vi "JOY_NORM.vi"(9 "Deadband":dbl, 11 "Joy Input":dbl) -> (3 "Joy Output":dbl)   [LabVIEW 2019]
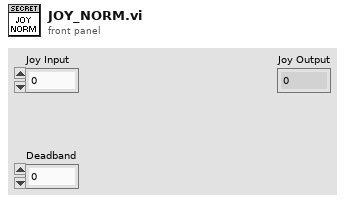
[diagram p1: front panel]
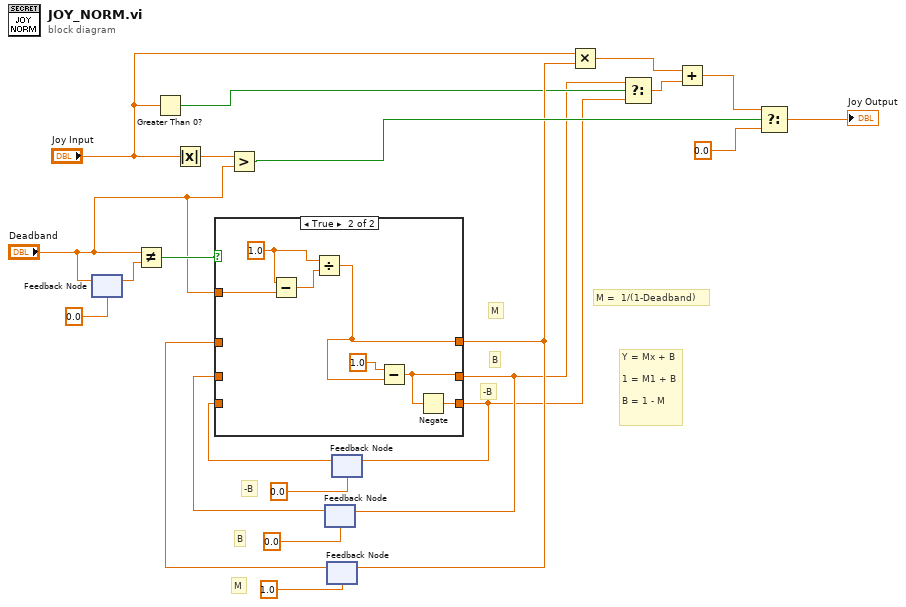
[diagram p0: block diagram]
diagram:
  # "-B"
  # "-B"
  # "M =  1/(1-Deadband)"
  # "Y = Mx + B\n\n1 = M1 + B\n\nB = 1 - M"
  # "M"
  # "B"
  # "B"
  # "M"
  n1 = feedback-in #1("Deadband") -> ()
  n2 = feedback #1(0.0 ("Deadband")) -> (w22:dbl)
  n3 = Not Equal?(x="Deadband", y=w22) -> (x != y?=w20:bool)
  n4 = Greater Than 0?(x="Joy Input") -> (x > 0?=w6:bool)
  n5 = Absolute Value(x="Joy Input") -> (abs(x)=w15:dbl)
  n6 = Greater?(x=w15, y="Deadband") -> (0:w13:bool)
  n7 = feedback #2(0.0 ("Deadband")) -> (w17:dbl)
  n8 = feedback #3(1.0 ("Deadband")) -> (w16:dbl)
  n9 = feedback #4(0.0 ("Deadband")) -> (w2:dbl)
  n10 = case shown="True" w20 {
    tunnel: w17 -> [w24 _]
    tunnel: [w24 w27] -> w5
    tunnel: w16 -> [w25 _]
    tunnel: [w25 w29] -> w11
    tunnel: "Deadband" -> [_ w30]
    tunnel: [w23 w26] -> w1
    tunnel: w2 -> [w23 _]
    frame False {
    }
    frame True {
      w31 = 1.0 ("x")
      n11 = Subtract(x=w31, y=w30) -> (x-y=w32:dbl)
      n12 = Divide(x=w31, y=w32) -> (x/y=w29:dbl)
      n13 = Subtract(x=1.0, y=w29) -> (x-y=w27:dbl)
      n14 = Negate(x=w27) -> (-x=w26:dbl)
    }
  }
  n15 = feedback-in #2(w5) -> ()
  n16 = feedback-in #3(w11) -> ()
  n17 = feedback-in #4(w1) -> ()
  n18 = Multiply(x="Joy Input", y=w11) -> (x*y=w10:dbl)
  n19 = Select(t=w5, s=w6, f=w1) -> (s? t:f=w8:dbl)
  n20 = Add(x=w10, y=w8) -> (x+y=w9:dbl)
  n21 = Select(t=w9, s=w13, f=0.0) -> (s? t:f=→"Joy Output":dbl)
